vi "Stop High-Speed Data Communication.vi"(8 "error in (no error)":errorcluster, 11 "Device ID (0)":i32) -> (0 "error out":errorcluster, 3 "Device ID out":i32)   [LabVIEW 2015, in "KEYENCE LJ-X8000A.lvlib"]
doc: "High-speed data communication will be terminated.\n\n<B>Note</B>:\nBuffered data will be maintained even if high-speed communication is stopped.\nIf high-speed communication is resumed, buffering will be executed after data of the same communication device is cleared."
uses:
  KEYENCE LJ-X8000A.lvlib
panel:
  # "(c) 2019 KEYENCE CORPORATION.  ALL RIGHTS RESERVED."
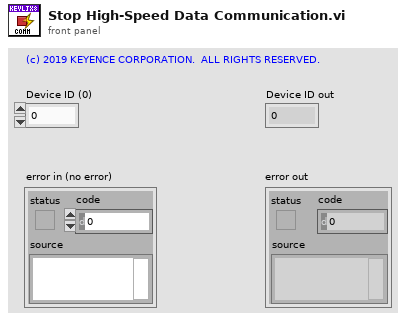
[diagram p1: front panel]
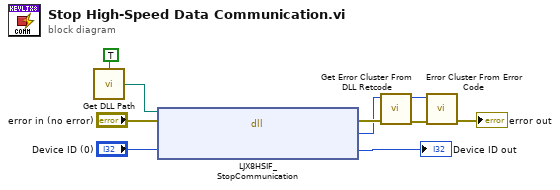
[diagram p0: block diagram]
diagram:
  n1 = call "Get DLL Path.vi"("isWrapperDLL (False)"=TRUE) -> ("DLL Path"=w6:path)  [unwired: 2 in]
  n2 = dll-call lib="C:/Program Files (x86)/National Instruments/LabVIEW 2018/instr.lib/KEYENCE LJ-X8000/LJX8_HighSpeedWrapper.*" fn="LJX8HSIF_StopCommunication"(path in=w6, error in="error in (no error)", "lDeviceId"="Device ID (0)") -> (error out=w4:errorcluster, "lRetCode"=w3:i32, "lDeviceId"=→"Device ID out":i32)  [unwired: 1 in, 1 out]
  n3 = call "Get Error Cluster From DLL Retcode.vi"("error in (no error)"=w4, "DLL Return Code"=w3) -> ("error out"=w5:errorcluster, "VI Error Code"=w1:i32)  [unwired: 8 in]
  n4 = call <vilib>:"Error Cluster From Error Code.vi"("error in (no error)"=w5, "error code (0)"=w1) -> ("error out"=→"error out":errorcluster)  [unwired: 7 in]
